vi "Timeout.vi"(0 "Interface In":refnum<class "TimedDoor_ITimerTimeout.lvclass">, 1 "TimeoutID":u32, 2 "TimeoutName":string, 5 "error in (no error)":errorcluster) -> (14 "Interface Out":refnum<class "TimedDoor_ITimerTimeout.lvclass">, 19 "error out":errorcluster)   [LabVIEW 2020, in "TimedDoor_ITimerTimeout.lvclass"]
uses:
  TimedDoor_ITimerTimeout.lvclass
  TimedDoor_ITimerTimeout.lvclass/TimedDoor_ITimerTimeout.ctl
  TimedDoor_class/TimedDoor.lvclass
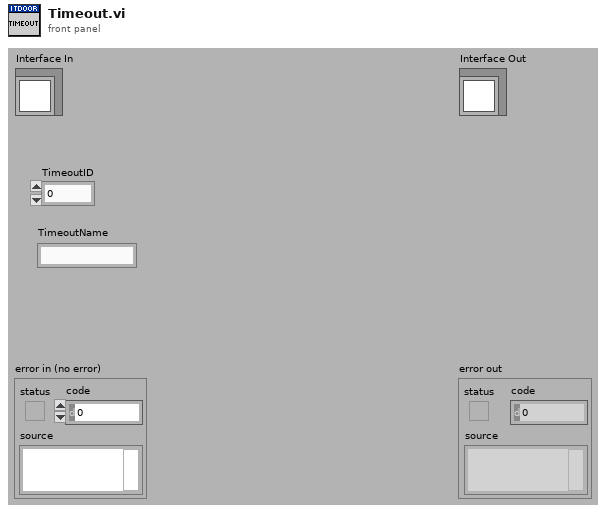
[diagram p1: front panel]
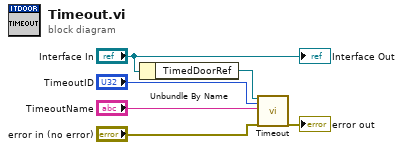
[diagram p0: block diagram]
diagram:
  n1 = Unbundle By Name("Interface In") -> ("TimedDoorRef"=w1:refnum<class "TimedDoor.lvclass">)
  n2 = call-dynamic "Timeout.vi"("reference in"=w1, "TimeoutID"="TimeoutID", "TimeoutName"="TimeoutName", "error in (no error)"="error in (no error)") -> ("error out"=→"error out":errorcluster)  [unwired: 14 in, 1 out]
  "Interface Out" <- "Interface In"
